vi "Periodic Tasks.vi"(8 "error in":errorcluster) -> ()   [LabVIEW 2017]
doc: "This VI runs in parallel to other tasks. It can contain as many user-defined periodic loops as you need. These can carry out PID or other sorts of timed response."
uses:
  <vilib>/Rock Robotics/SystemInterfaces/AI/FPGA_AIChannel.ctl
  <vilib>/Rock Robotics/WPI/Accelerometer/WPI_AccelerometerRange.ctl
  <vilib>/Rock Robotics/WPI/Utilities/WPI_GetSetVariantRefNum.vi
  <vilib>/Rock Robotics/Network Tables/NT Write Number.vi
  <vilib>/Rock Robotics/WPI/Ultrasonic/WPI_SonarMB1010AnalogGetRange.vi
  <vilib>/Rock Robotics/WPI/Ultrasonic/WPI_SonarMB1010AnalogRefNum Registry Set.vi
  <vilib>/Rock Robotics/WPI/Ultrasonic/WPI_SonarMB1010AnalogOpen.vi
  <vilib>/Rock Robotics/WPI/Ultrasonic/WPI_SonarMB1010AnalogClose.vi
  <vilib>/Rock Robotics/WPI/Accelerometer/InternalAccelerometer/WPI_AccelerometerInternalOpen.vi
  <vilib>/Rock Robotics/Network Tables/NT Write Boolean.vi
  <vilib>/Rock Robotics/Network Tables/NT Read Boolean.vi
panel:
  in  "Scaling Factor":dbl=0.025
  in  "Average Bits":u8=3 max=15
  out "distance":dbl(slide)=125.0 scale=0.0..250.0 scale format="%3d"
  out "error out":errorcluster
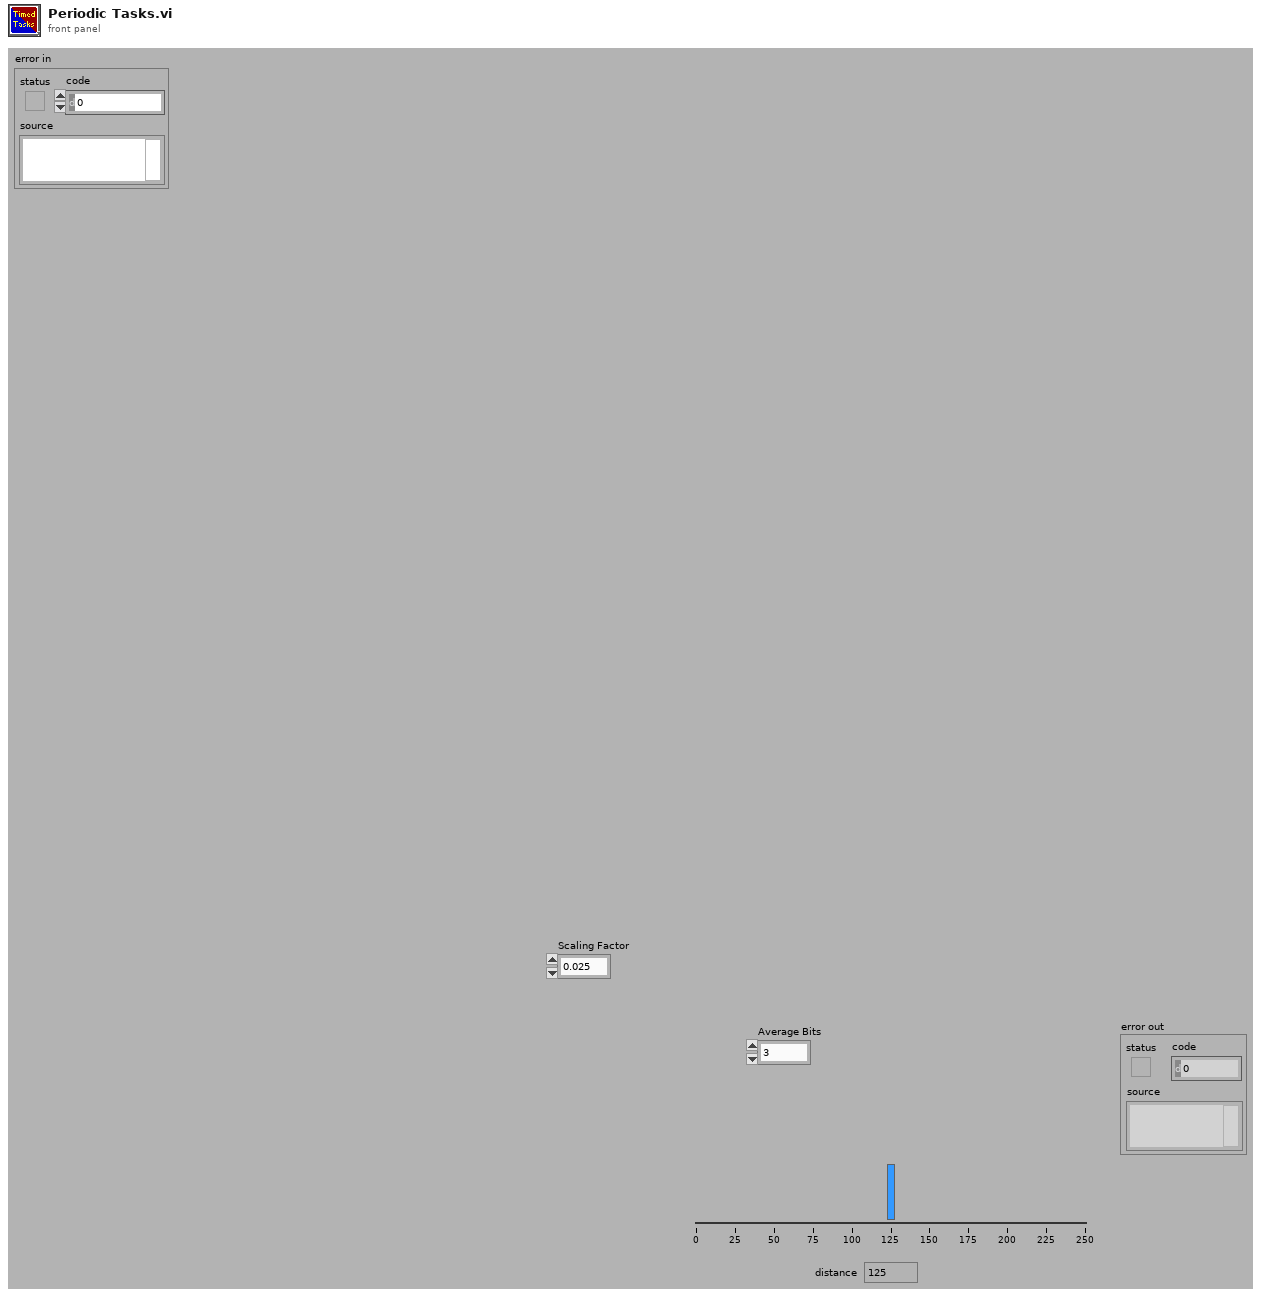
[diagram p1: front panel]
types:
  T1 = typedef "WPI_AccelerometerRange.ctl" = enum16{"+/- 2 g", "+/- 4 g", "+/- 8 g"}
  T2 = typedef "FPGA_AIChannel.ctl" = enum8{"AI 0", "AI 1", "AI 2", "AI 3", "AI MXP 0", "AI MXP 1", "AI MXP 2", "AI MXP 3", "Invalid"}
  T3 = typedef "WPI_AccelerometerDevRef.ctl" = cluster{"DevStatus":errorcluster, "Scaling":T4, "Analog Channels":T5, "I2C Bus":T6, "SPI Bus":T7, "Accel Range":T8, "ADXL Axes":T9, "Handle":i32, "Device Address":u8, "Accel Type":enum16{"Analog", "ADXL345 I2C", "ADXL345 SPI", "Internal", "ADXL362 SPI"}}
  T4 = typedef "WPI_AccelerometerScaling.ctl" = cluster{"Gain (VoltsPerG)":dbl, "Center Voltage":dbl}
  T5 = typedef "WPI_AccelerometerAnalogChannels.ctl" = cluster{"X-Axis":T2, "Y-Axis":T2, "Z-Axis":T2}
  T6 = typedef "i2c_bus.ctl" = enum16{"I2C On-Board", "I2C MXP", "Invalid"}
  T7 = typedef "spi_bus.ctl" = enum16{"SPI On-Board, CS0", "SPI On-Board, CS1", "SPI On-Board, CS2", "SPI On-Board, CS3", "SPI MXP", "Invalid"}
  T8 = typedef "ADXL345 Range.ctl" = u8
  T9 = typedef "WPI_AccelerometerADXL345 Axes.ctl" = cluster{"X-Axis":bool, "Y-Axis":bool, "Z-Axis":bool}
  T10 = typedef "WPI_RobotDriveDevRef.ctl" = cluster{"DevStatus":errorcluster, "Motors[]":T11[], "Square Inputs":bool, "Max Output":dbl}
  T11 = typedef "WPI_MotorControlDeviceRef.ctl" = cluster{"DeviceStatus":errorcluster, "Type":T12, "PWM":cluster{"PWM Channel":T13, "DeadBand":T14}, "CAN":cluster{"Device Number":u8, "SetOutput VI Ref":variant, "GetOutput VI Ref":variant, "Enable VI Ref":variant, "Disable VI Ref":variant, "Data":variant}, "Invert":bool, "DIO PWM":cluster{"PWM \"Enable\" Channel":T13, "DIOChannel":T15, "PWM Rate":dbl}}
  T12 = typedef "WPI_MotorControlType.ctl" = enum16{"PWM", "CAN", "DIO PWM"}
  T13 = typedef "FPGA_DIOPWMChannel.ctl" = enum8{"PWM 0", "PWM 1", "PWM 2", "PWM 3", "PWM 4", "PWM 5", "PWM 6", "PWM 7", "PWM 8", "PWM 9", "PWM MXP 0", "PWM MXP 1", "PWM MXP 2", "PWM MXP 3", "PWM MXP 4", "PWM MXP 5", "PWM MXP 6", "PWM MXP 7", "PWM MXP 8", "PWM MXP 9", "Invalid"}
  T14 = typedef "WPI_PWMDeadband.ctl" = cluster{"Name":string, "maxPositivePwm":i32, "minPositivePwm":i32, "centerPwm":i32, "maxNegativePwm":i32, "minNegativePwm":i32, "angularRange":u16}
  T15 = typedef "FPGA_DIOChannel.ctl" = enum8{"DIO 0", "DIO 1", "DIO 2", "DIO 3", "DIO 4", "DIO 5", "DIO 6", "DIO 7", "DIO 8", "DIO 9", "DIO MXP 0", "DIO MXP 1", "DIO MXP 2", "DIO MXP 3", "DIO MXP 4", "DIO MXP 5", "DIO MXP 6", "DIO MXP 7", "DIO MXP 8", "DIO MXP 9", "DIO MXP 10", "DIO MXP 11", "DIO MXP 12", "DIO MXP 13", "DIO MXP 14", "DIO MXP 15", "SPI Port CS1", "SPI Port CS2", "SPI Port CS3", "SPI Port MISO", "SPI Port MOSI", "Invalid"}
  T16 = typedef "WPI_JoystickDevRef.ctl" = cluster{"Device":T17}
  T17 = typedef "WPI_JoystickDeviceEnum.ctl" = enum16{"USB 0", "USB 1", "USB 2", "USB 3", "USB 4", "USB 5"}
  T18 = cluster{"JoystickDevRef":T16, "RobotDriveDevRef":T10}
  T19 = typedef "WPI_GyroDevRef.ctl" = cluster{"DevStatus":errorcluster, "Analog Channel":T2, "Gain (VoltsPerDegree/Second)":dbl, "Gyro Type":enum16{"Analog", "XRS450"}, "Handle":i32, "SPI Bus":T7, "Device Found":bool, "Sample Rate":dbl, "Calibrate On Open":bool, "Offset":dbl}
  T20 = cluster{"X-Axis":dbl, "Y-Axis":dbl, "Z-Axis":dbl}
  T21 = typedef "WPI_SonarMB1010AnalogDeviceRef.ctl" = cluster{"AIDeviceRef":T22, "Scaling factor (V/in)":dbl, "Average Bits":u8}
  T22 = typedef "WPI_AnalogChannelDevRef.ctl" = cluster{"DevStatus":errorcluster, "Analog Channel":T2}
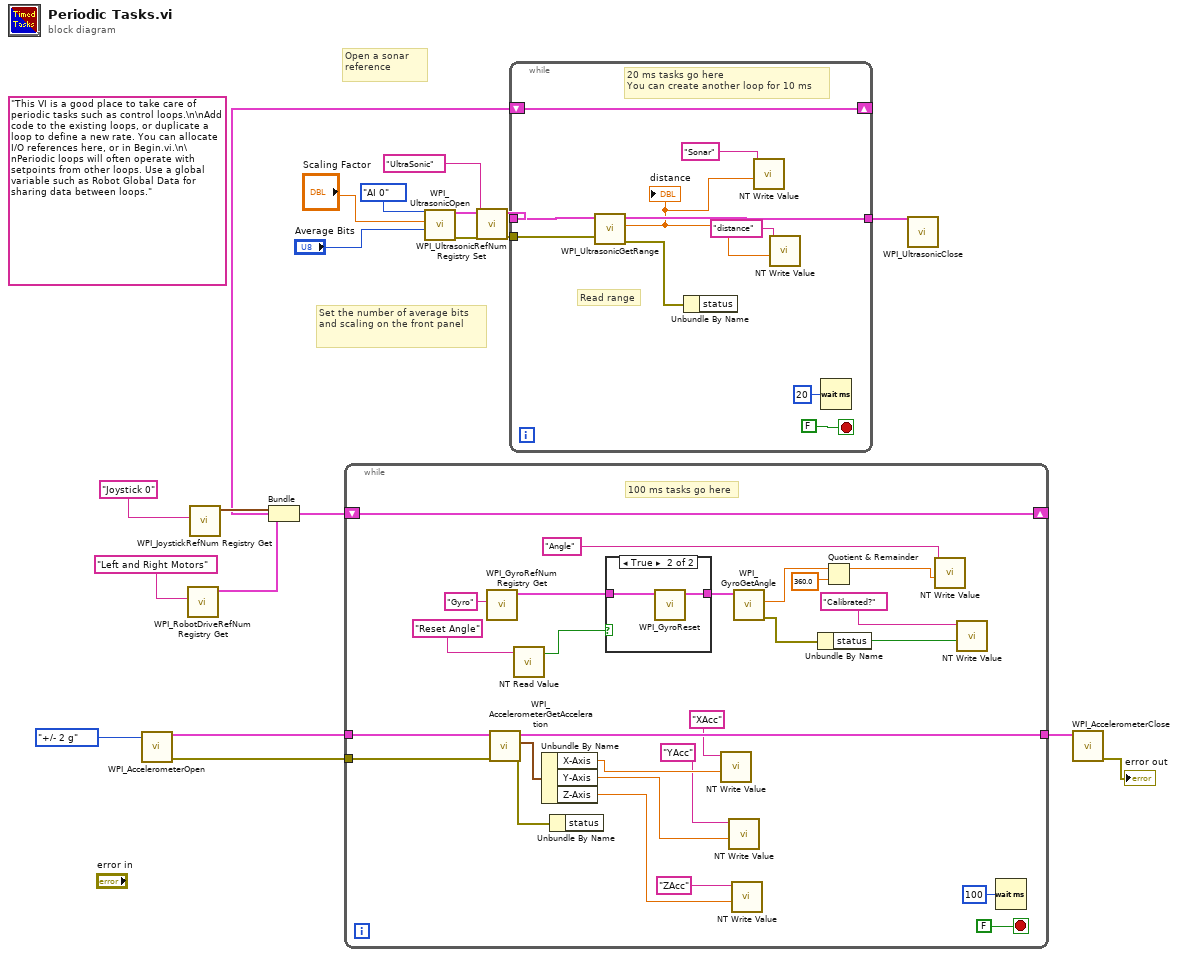
[diagram p0: block diagram]
diagram:
  (unwired) "This VI is a good place to take care of periodic tasks such as control loops.\n\nAdd code to the existing loops, or duplicate a loop to define a new rate. You can allocate I/O references here, or in Begin.vi.\n\nPeriodic loops will often operate with setpoints from other loops. Use a global variable such as Robot Global Data for sharing data between loops."
  # "Set the number of average bits and scaling on the front panel"
  # "Open a sonar reference"
  n1 = call-poly <vilib>:"WPI_AccelerometerOpen.vi"("Accel Range"=WPI_AccelerometerRange."+/- 2 g") -> ("error out"=w13:errorcluster, "AccelerometerDevRef"=w14:T3)  [unwired: 9 in]
  n2 = call <vilib>:"WPI_RobotDriveRefNum Registry Get.vi"("refnum name"="Left and Right Motors") -> ("RobotDriveDevRef"=w16:T10)  [unwired: 1 in, 9 out]
  n3 = call <vilib>:"WPI_JoystickRefNum Registry Get.vi"("refnum name"="Joystick 0") -> ("JoystickDevRef"=w17:T16)  [unwired: 1 in, 9 out]
  n4 = Bundle("JoystickDevRef"=w17, "RobotDriveDevRef"=w16) -> (w15:T18)  [unwired: 1 out]
  n5 = while {
    shift-right: [w43] -> _
    shift-left: w15 -> [w43]
    tunnel: w14 -> [w28]
    tunnel: w13 -> [w27]
    tunnel: [w26] -> w11
    stop <- FALSE stop-if-true
    # "100 ms tasks go here"
    n6 = call <vilib>:"WPI_GyroRefNum Registry Get.vi"("refnum name"="Gyro") -> ("GyroDevRef"=w36:T19)  [unwired: 9 in, 1 out]
    n7 = call <vilib>:"WPI_AccelerometerGetAcceleration.vi"("error in"=w27, "AccelerometerDevRef"=w28) -> ("error out"=w29:errorcluster, "Accelerations"=w30:T20, "AccelerometerDevRef"=w26:T3)  [unwired: 7 in]
    n8 = call-poly <vilib>:"NT Read Value.vi"("Name"="Reset Angle") -> ("Boolean"=w39:bool)  [unwired: 9 in, 1 out]
    n9 = Unbundle By Name(w30) -> ("X-Axis"=w25:dbl, "Y-Axis"=w24:dbl, "Z-Axis"=w23:dbl)
    n10 = Unbundle By Name(w29) -> ()  [unwired: 1 out]
    n11 = case shown="True" w39 {
      tunnel: [w46 w48] -> w32
      tunnel: w36 -> [w46 w47]
      frame False {
      }
      frame True {
        n12 = call <vilib>:"WPI_GyroReset.vi"("GyroDevRef"=w47) -> ("GyroDevRef"=w48:T19)  [unwired: 9 in, 1 out]
      }
    }
    n13 = call-poly <vilib>:"NT Write Value.vi"("Numeric"=w25, "Name"="XAcc") -> ()  [unwired: 9 in, 1 out]
    n14 = call-poly <vilib>:"NT Write Value.vi"("Numeric"=w24, "Name"="YAcc") -> ()  [unwired: 9 in, 1 out]
    n15 = call-poly <vilib>:"NT Write Value.vi"("Numeric"=w23, "Name"="ZAcc") -> ()  [unwired: 9 in, 1 out]
    n16 = call <vilib>:"WPI_GyroGetAngle.vi"("GyroDevRef"=w32) -> ("error out"=w34:errorcluster, "Angle"=w33:dbl)  [unwired: 6 in, 3 out]
    n17 = Unbundle By Name(w34) -> ("status"=w42:bool)
    n18 = Quotient & Remainder(x=w33, y=360.0) -> (x-y*floor(x/y)=w37:dbl)  [unwired: 1 out]
    n19 = call-poly <vilib>:"NT Write Value.vi"("Numeric"=w37, "Name"="Angle") -> ()  [unwired: 9 in, 1 out]
    n20 = call-poly <vilib>:"NT Write Value.vi"("Boolean"=w42, "Name"="Calibrated?") -> ()  [unwired: 9 in, 1 out]
    n21 = Wait (ms)(milliseconds to wait=u32 100) -> ()  [unwired: 1 out]
  }
  n22 = call-poly <vilib>:"WPI_UltrasonicOpen.vi"("Average Bits"="Average Bits", "Scaling factor (V/in)"="Scaling Factor", "Analog Channel"=FPGA_AIChannel."AI 0") -> ("error out"=w6:errorcluster, "SonarMB1010AnalogDevRef"=w4:T21)  [unwired: 7 in]
  n23 = call-poly <vilib>:"WPI_UltrasonicRefNum Registry Set.vi"("error in (no error)"=w6, "refnum name"="UltraSonic", "SonarMB1010AnalogDevRef"=w4) -> ("error out"=w2:errorcluster, "SonarMB1010AnalogDevRef"=w3:T21)  [unwired: 7 in]
  n24 = while {
    shift-right: [w56] -> _
    shift-left: w15 -> [w56]
    tunnel: [w54] -> w10
    tunnel: w3 -> [w53]
    tunnel: w2 -> [w49]
    stop <- FALSE stop-if-true
    # "Read range"
    # "20 ms tasks go here\nYou can create another loop for 10 ms"
    n25 = call-poly <vilib>:"WPI_UltrasonicGetRange.vi"("error in"=w49, "SonarMB1010AnalogDevRef"=w53) -> ("error out"=w55:errorcluster, "Distance"=w51:dbl, "SonarMB1010AnalogDevRef"=w54:T21)  [unwired: 7 in]
    "distance" <- w51
    n26 = Unbundle By Name(w55) -> ()  [unwired: 1 out]
    n27 = call-poly <vilib>:"NT Write Value.vi"("Numeric"=w51, "Name"="Sonar") -> ()  [unwired: 9 in, 1 out]
    n28 = call-poly <vilib>:"NT Write Value.vi"("Numeric"=w51, "Name"="distance") -> ()  [unwired: 9 in, 1 out]
    n29 = Wait (ms)(milliseconds to wait=u32 20) -> ()  [unwired: 1 out]
  }
  n30 = call-poly <vilib>:"WPI_UltrasonicClose.vi"("SonarMB1010AnalogDevRef"=w10) -> ()  [unwired: 10 in, 1 out]
  n31 = call <vilib>:"WPI_AccelerometerClose.vi"("AccelerometerDevRef"=w11) -> ("error out"=→"error out":errorcluster)  [unwired: 10 in]
